vi "Start Acquisition.vi"(8 "error in (no error)":errorcluster, 10 "Threshold":dbl, 11 "Supervisor in":refnum<class "Supervisor.lvclass">) -> (0 "error out":errorcluster, 3 "Supervisor out":refnum<class "Supervisor.lvclass">)   [LabVIEW 2020, in "Supervisor.lvlib" / "Supervisor.lvclass"]
uses:
  Supervisor.lvclass
  Supervisor.lvclass/Supervisor.ctl
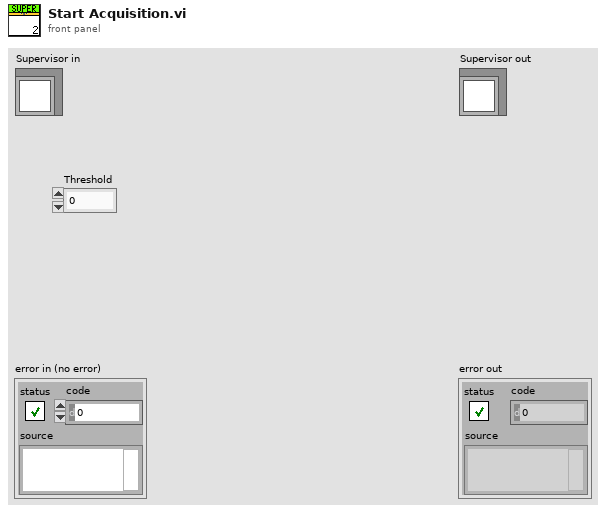
[diagram p1: front panel]
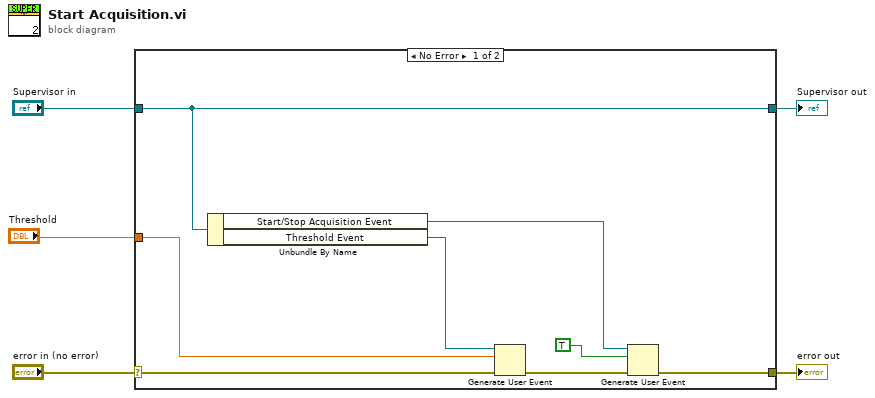
[diagram p0: block diagram]
diagram:
  n1 = case shown="No Error" "error in (no error)" {
    selector: "error in (no error)" -> [w13 w15]
    tunnel: [w6 w15] -> w4
    tunnel: [w12 w14] -> w2
    tunnel: "Supervisor in" -> [w12 w14]
    tunnel: "Threshold" -> [w10 _]
    frame No Error {
      n2 = Unbundle By Name(w12) -> ("Start/Stop Acquisition Event"=w8:refnum<user-event>, "Threshold Event"=w11:refnum<user-event>)
      n3 = Generate User Event(user event=w11, event data cluster=w10, error in=w13) -> (error out=w7:errorcluster)  [unwired: 1 in, 1 out]
      n4 = Generate User Event(user event=w8, event data cluster=TRUE ("event data"), error in=w7) -> (error out=w6:errorcluster)  [unwired: 1 in, 1 out]
    }
    frame Error {
    }
  }
  "error out" <- w4
  "Supervisor out" <- w2
